vi "Simple Add.vi"() -> ()   [LabVIEW 2017]
panel:
  out "Sum":dbl
  in  "Addend 3":dbl
  in  "Addend 2":dbl
  in  "Addend 1":dbl
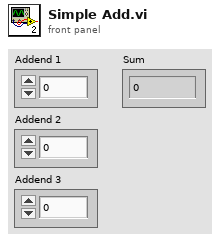
[diagram p1: front panel]
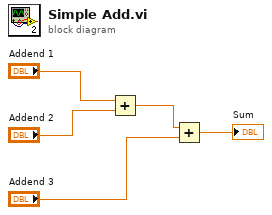
[diagram p0: block diagram]
diagram:
  n1 = Add(x="Addend 1", y="Addend 2") -> (x+y=w5:dbl)
  n2 = Add(x=w5, y="Addend 3") -> (x+y=→"Sum":dbl)
